vi "UNDT_StringToData(SubVI).vi"(5 "UNDT_Cluster 3":T1 {"Gain Coeff" format="%#_6e"; "Reserve 1" format="%02x"; "Mux TX/RX" format="%02x"; "ScanDelay" format="%02x"; "PacketCounter" format="%08x"; "SamplingInterval" format="%#_6e"; "Lose Packet" format="%08x"; "EncodersParam2" format="%016x"; "EncodersParam1" format="%016x"; "CRC 8" format="%02x"; "N chanel" format="%02x"; "N tick" format="%02x"; "Ncycle" format="%04x"; "FrameFormatVersion" format="%02x"; "MagicWord" format="%.0x"}, 7 "OptionPACK5":T2={"MagicWordStr"="xV4\u0012", "Header size"=56, "Проверка CRC8"=TRUE, "Проверка конца пакета"=FALSE, "GainCompens"=FALSE, "Неотбрасывать BadEnd пакеты"=TRUE, "Неотбрасывать BadCRC пакеты"=TRUE, "Привести к 1"=FALSE, "GainCoef"=FALSE, "K_scale"=0.0, "ScaleOrdinate"=enum."Проценты"}, 10 "SkipSample":i32=100, 11 "string in":string) -> (1 "Over":bool, 2 "DataOut":dbl[](array[numeric]) format="%_3p")   [LabVIEW 2017]
uses:
  Control_EU/OptionPACK5.ctl
  Control_EU/UNDT_ClusterPackRevers (Type).ctl
panel:
  out "x*y":dbl
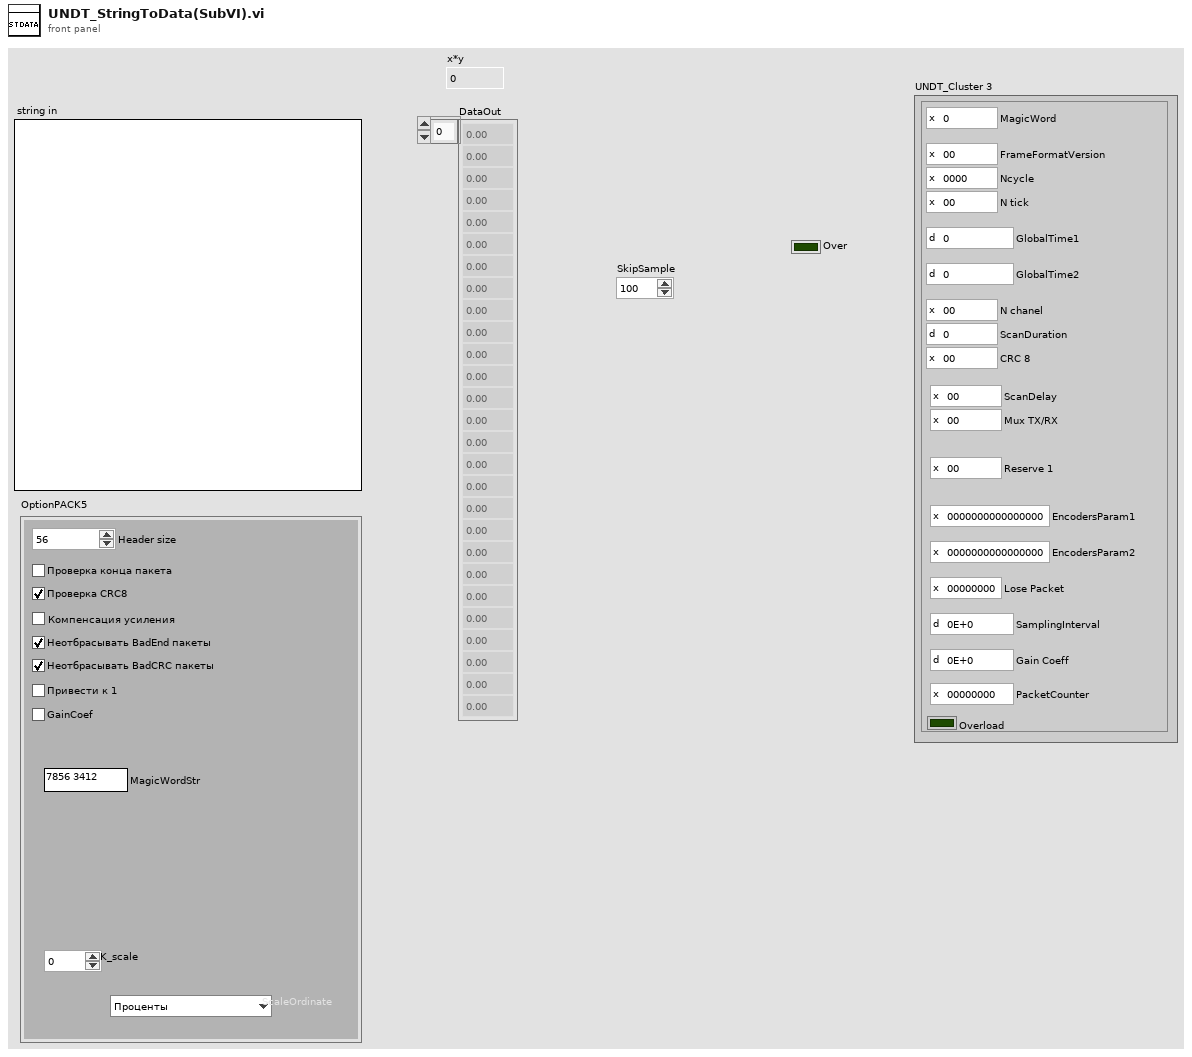
[diagram p1: front panel]
types:
  T1 = typedef "UNDT_ClusterPackRevers (Type).ctl" = cluster{"PacketCounter":u32, "Gain Coeff":sgl, "SamplingInterval":sgl, "Lose Packet":u32, "EncodersParam2":u64, "EncodersParam1":u64, "Reserve 1":u8, "Mux TX/RX":u8, "ScanDelay":u16, "CRC 8":u8, "ScanDuration":u16, "N chanel":u8, "GlobalTime2":u32, "GlobalTime1":u32, "N tick":u8, "Ncycle":u16, "FrameFormatVersion":u8, "MagicWord":u32, "Overload":bool}
  T2 = typedef "OptionPACK5.ctl" = cluster{"MagicWordStr":string, "Header size":u32, "Проверка CRC8":bool, "Проверка конца пакета":bool, "GainCompens":bool, "Неотбрасывать BadEnd пакеты":bool, "Неотбрасывать BadCRC пакеты":bool, "Привести к 1":bool, "GainCoef":bool, "K_scale":dbl, "ScaleOrdinate":enum16{"Отсчеты АЦП (±32767)", "Проценты", "Вольты", "дБмкВ (отн. 1 мкВ)", "Отсчеты АЦП (±1)"}}
  T3 = enum16{"Отсчеты АЦП (±32767)", "Проценты", "Вольты", "дБмкВ (отн. 1 мкВ)", "Отсчеты АЦП (±1)"}
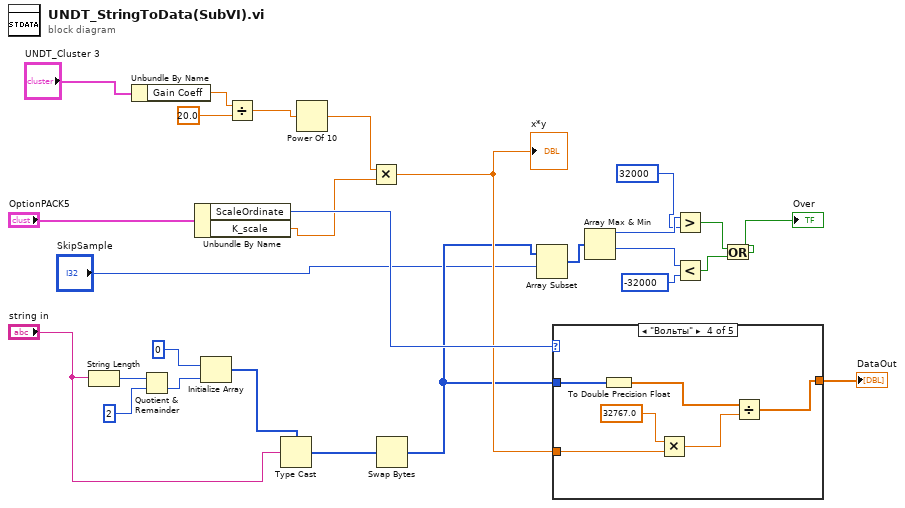
[diagram p0: block diagram]
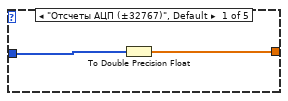
[diagram p2: hidden frame]
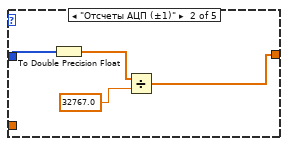
[diagram p3: hidden frame]
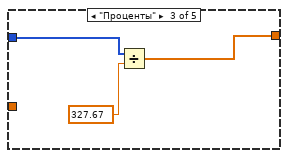
[diagram p4: hidden frame]
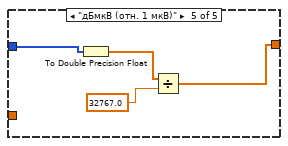
[diagram p5: hidden frame]
diagram:
  n1 = String Length(string="string in") -> (length=w27:i32)
  n2 = Unbundle By Name("UNDT_Cluster 3") -> ("Gain Coeff"=w16:sgl)
  n3 = Quotient & Remainder(x=w27, y=2) -> (floor(x/y)=w24:i32)  [unwired: 1 out]
  n4 = Unbundle By Name("OptionPACK5") -> ("ScaleOrdinate"=w18:T3, "K_scale"=w13:dbl)
  n5 = Initialize Array(i16 0 ("n"), w24) -> (w21:i16[])
  n6 = Divide(x=w16, y=sgl 20.0) -> (x/y=w14:sgl)
  n7 = Type Cast(type=w21, x="string in") -> (*(type *) &x=w22:i16[])
  n8 = Power Of 10(x=w14) -> (10^x=w12:sgl)
  n9 = Multiply(x=w12, y=w13) -> (x*y=w11:dbl)
  "x*y" <- w11
  n10 = Swap Bytes(anything=w22) -> (byte swapped=w3:i16[])
  n11 = Array Subset(array=w3, index="SkipSample") -> (w1:i16[])  [unwired: 1 in]
  n12 = case shown="\"Вольты\"" w18 {
    tunnel: w3 -> [w29 w33 w36 w41 w44]
    tunnel: [w28 w30 w35 w40 w43] -> w25
    tunnel: w11 -> [_ _ _ w37 _]
    frame "Отсчеты АЦП (±32767)", Default {
      n13 = To Double Precision Float(number=w29) -> (double precision float=w28:dbl[])
    }
    frame "Отсчеты АЦП (±1)" {
      n14 = To Double Precision Float(number=w33) -> (double precision float=w31:dbl[])
      n15 = Divide(x=w31, y=32767.0) -> (x/y=w30:dbl[])
    }
    frame "Проценты" {
      n16 = Divide(x=w36, y=327.67) -> (x/y=w35:dbl[])
    }
    frame "Вольты" {
      n17 = To Double Precision Float(number=w41) -> (double precision float=w42:dbl[])
      n18 = Multiply(x=32767.0 ("y"), y=w37) -> (x*y=w38:dbl)
      n19 = Divide(x=w42, y=w38) -> (x/y=w40:dbl[])
    }
    frame "дБмкВ (отн. 1 мкВ)" {
      n20 = To Double Precision Float(number=w44) -> (double precision float=w45:dbl[])
      n21 = Divide(x=w45, y=32767.0) -> (x/y=w43:dbl[])
    }
  }
  "DataOut" <- w25
  n22 = Array Max & Min(array=w1) -> (max value=w10:i16, min value=w8:i16)  [unwired: 2 out]
  n23 = Greater?(x=w10, y=i16 32000 ("n")) -> (0:w5:bool)
  n24 = Less?(x=w8, y=i16 -32000 ("n")) -> (x < y?=w6:bool)
  n25 = Or(x=w5, y=w6) -> (x .or. y?=→"Over":bool)
